vi "refNewton Ralphson Zero Finder.vi"   [LabVIEW 2017, in "NI_Gmath.lvlib"]
uses:
  <vilib>/gmath/NI_Gmath.lvlib
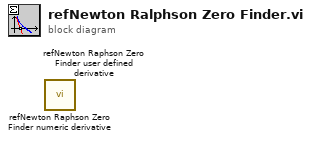
[diagram p0: block diagram]
diagram:
  n1 = call <vilib>:"refNewton Raphson Zero Finder numeric derivative.vi"() -> ()  [unwired: 8 in, 4 out]
  n2 = call <vilib>:"refNewton Raphson Zero Finder user defined derivative.vi"() -> ()  [unwired: 8 in, 4 out]
